vi "Get Text.vi"(8 "error in (no error)":errorcluster, 11 "ScintillaNET in":refnum<class "ScintillaNET.lvclass">) -> (0 "error out":errorcluster, 2 "Text":string, 3 "ScintillaNET out":refnum<class "ScintillaNET.lvclass">)   [LabVIEW 2018, in "ScintillaNET.lvclass"]
uses:
  ScintillaNET.lvclass
  ScintillaNET.lvclass/ScintillaNET.ctl
  D:/project/hobby/LF2R/LabVIEW/source/ScintillaNET/dll/ScintillaNET.dll
  dll/ScintillaNET.dll
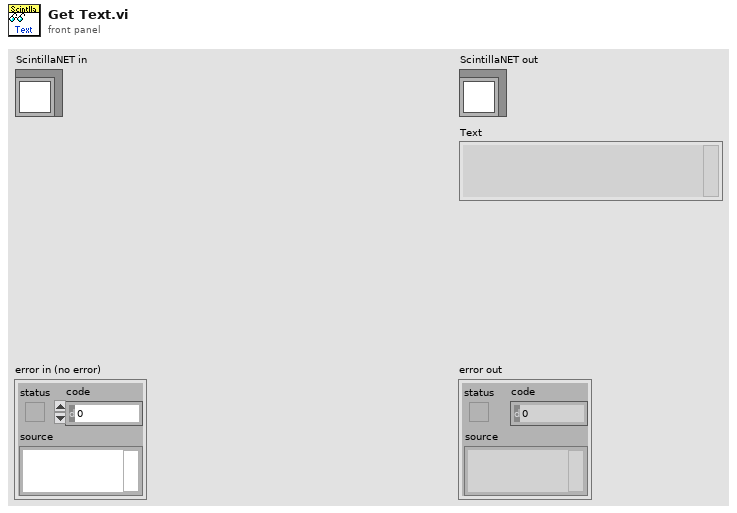
[diagram p1: front panel]
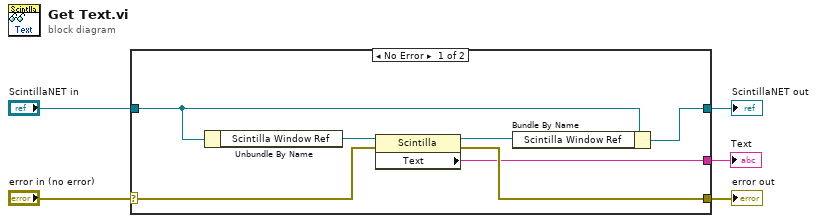
[diagram p0: block diagram]
diagram:
  n1 = case shown="No Error" "error in (no error)" {
    selector: "error in (no error)" -> [w11 w14]
    tunnel: [w10 w14] -> w4
    tunnel: [w12 w13] -> w2
    tunnel: "ScintillaNET in" -> [w8 w13]
    tunnel: [w6 _] -> w1
    frame No Error {
      n2 = Unbundle By Name(w8) -> ("Scintilla Window Ref"=w7:refnum<k24>)
      n3 = property class="Scintilla"(reference=w7, error in=w11) -> (reference out=w9:refnum<k24>, error out=w10:errorcluster, "Text"=w6:string)
      n4 = Bundle By Name(cluster=w8, "Scintilla Window Ref"=w9) -> (w12:refnum<class "ScintillaNET.lvclass">)
    }
    frame Error {
    }
  }
  "error out" <- w4
  "ScintillaNET out" <- w2
  "Text" <- w1
